vi "subComputeDependencyListSubsetParams.vi"(7 "size":i32, 10 "length (-1)":i32=-1, 11 "index":i32) -> (2 "length out":i32, 3 "index out":i32)   [LabVIEW 2020, in "SolutionBuilder.lvlib" / "BuildManager.lvclass"]
uses:
  BuildManager.lvclass
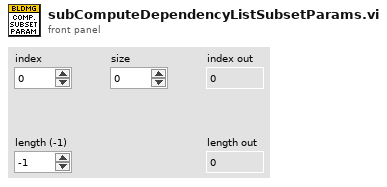
[diagram p1: front panel]
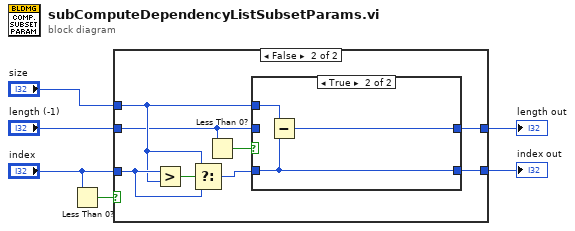
[diagram p0: block diagram]
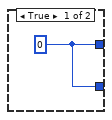
[diagram p2: hidden frame]
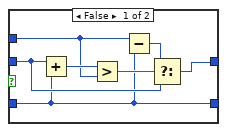
[diagram p3: hidden frame]
diagram:
  n1 = Less Than 0?(x="index") -> (x < 0?=w1:bool)
  n2 = case shown="False" w1 {
    tunnel: "index" -> [_ w12]
    tunnel: "length (-1)" -> [_ w9]
    tunnel: "size" -> [_ w11]
    tunnel: [w7 w15] -> w6
    tunnel: [w7 w14] -> w5
    frame True {
      w7 = 0 ("length (-1)")
    }
    frame False {
      n3 = Greater?(x=w12, y=w11) -> (0:w13:bool)
      n4 = Select(t=w11, s=w13, f=w12) -> (s? t:f=w8:i32)
      n5 = Less Than 0?(x=w9) -> (x < 0?=w10:bool)
      n6 = case shown="True" w10 {
        tunnel: w11 -> [w18 w23]
        tunnel: w8 -> [w16 w25]
        tunnel: [w16 w25] -> w15
        tunnel: w9 -> [w19 _]
        tunnel: [w21 w24] -> w14
        frame False {
          n7 = Add(x=w19, y=w16) -> (x+y=w20:i32)
          n8 = Greater?(x=w20, y=w18) -> (0:w22:bool)
          n9 = Subtract(x=w18, y=w16) -> (x-y=w17:i32)
          n10 = Select(t=w17, s=w22, f=w19) -> (s? t:f=w21:i32)
        }
        frame True {
          n11 = Subtract(x=w23, y=w25) -> (x-y=w24:i32)
        }
      }
    }
  }
  "index out" <- w6
  "length out" <- w5
